vi "Execute.vi"(8 "Error In":errorcluster, 9 "Workspace":T1, 10 "Control In":T2, 11 "Dispense in":refnum<class "Dispense.lvclass">) -> (0 "Error Out":errorcluster, 2 "Control Out":T2, 3 "Dispense in 2":refnum<class "Dispense.lvclass">)   [LabVIEW 2020, in "Dispense.lvclass"]
uses:
  Dispense.lvclass
  Controller/Controllers.ctl
  Controller/I-O/I-O.lvclass
  Controller/Dispenser/Dispenser.lvclass
  C:/Program Files (x86)/Aerotech/A3200/LabVIEW/2010/Bin/Aerotech.A3200.dll
  Program Files (x86)/Aerotech/A3200/LabVIEW/2010/Bin/Aerotech.A3200.dll
  Workspace/Workspace.ctl
  Dispense.lvclass/Dispense.ctl
  Controller/Motion/Motion.lvclass
  Controller/Motion/A3200/A3200.lvclass
  Controller/Controller.lvclass
  Workspace/Fixture.lvclass
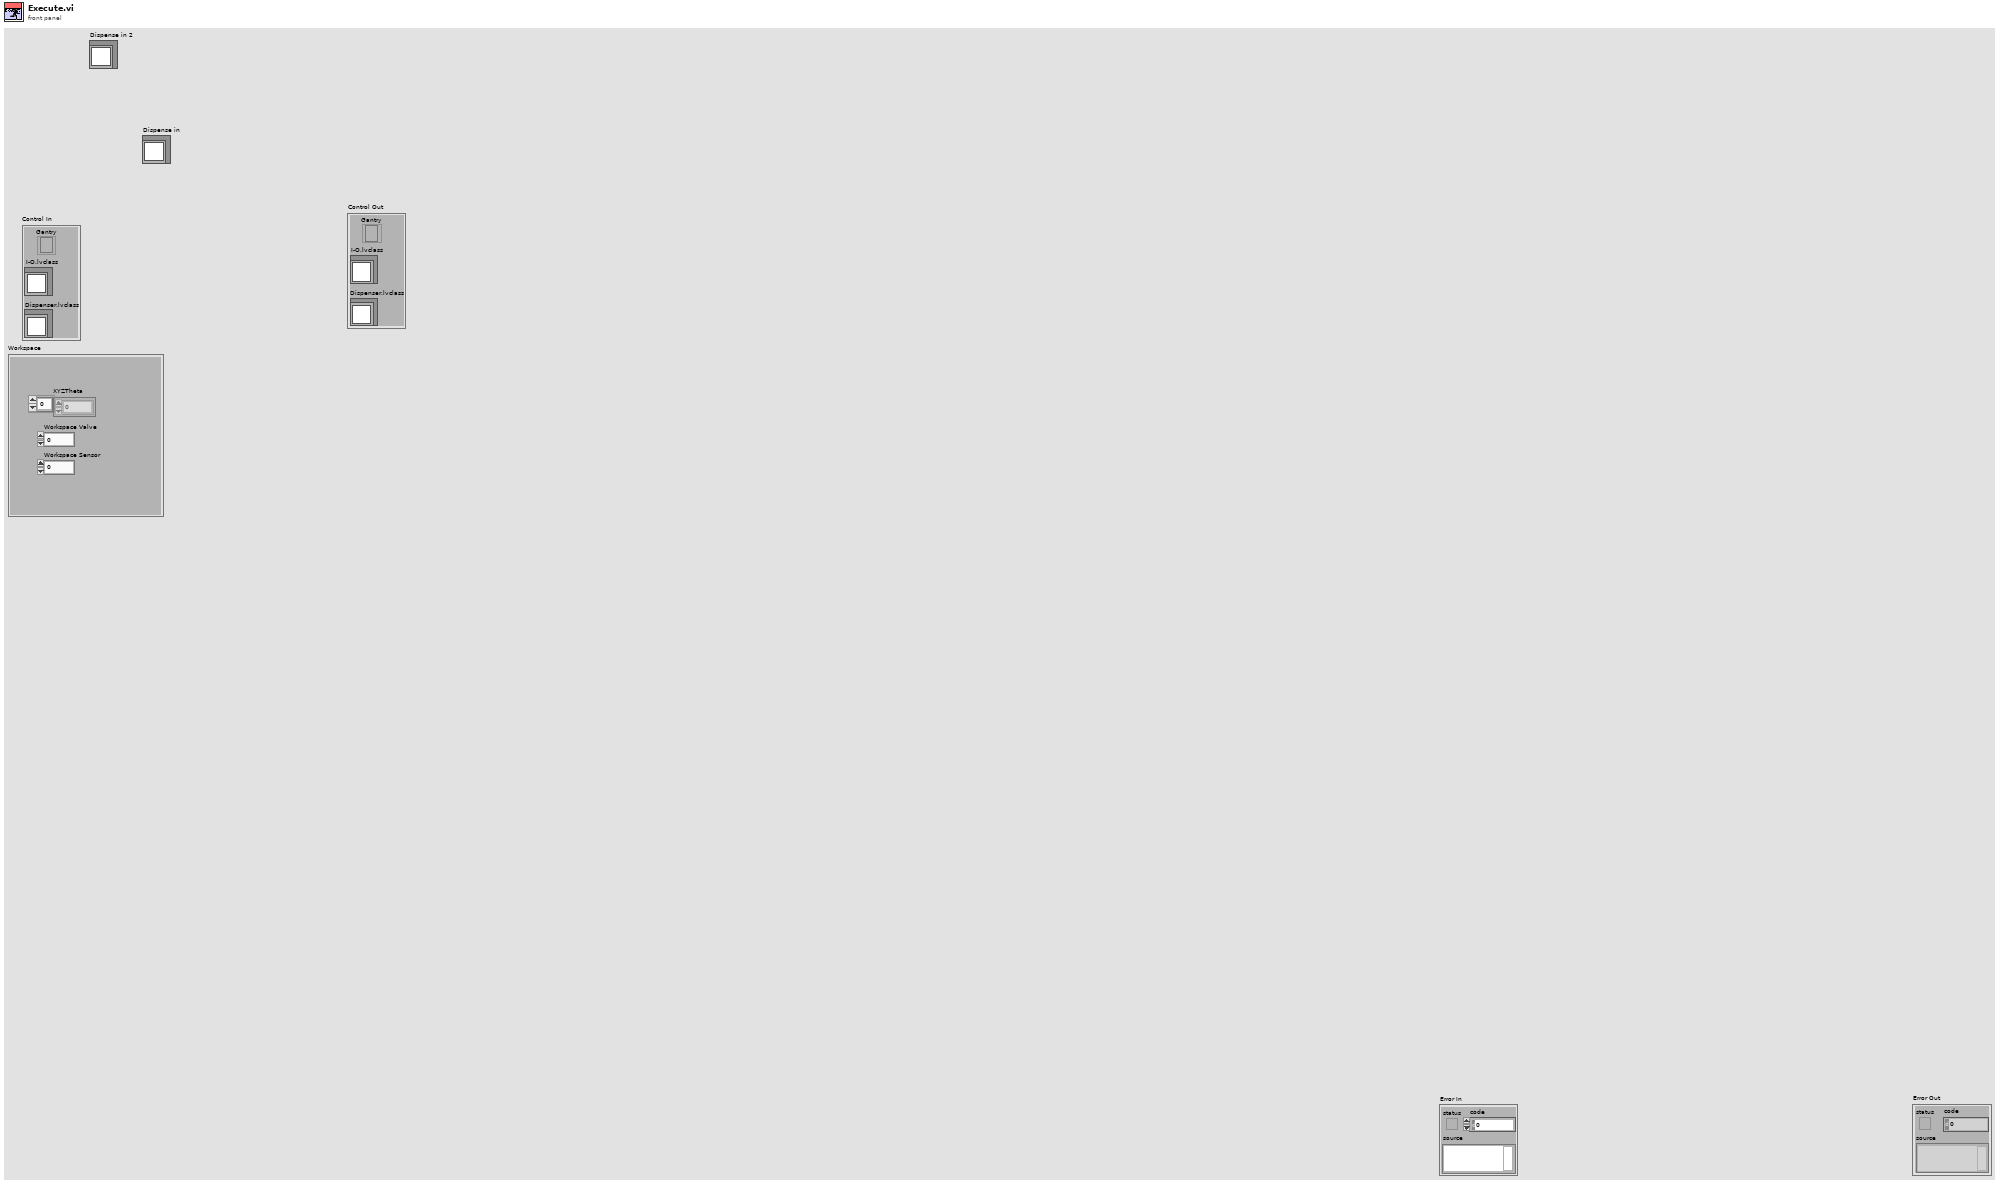
[diagram p1: front panel]
types:
  T1 = typedef "Fixture.lvclass/Workspace.ctl" = cluster{"XYZTheta":dbl[], "Workspace Valve":i32, "Workspace Sensor":i32}
  T2 = typedef "Controller.lvclass/Controllers.ctl" = cluster{"I-O.lvclass":refnum<class "I-O.lvclass">, "Dispenser.lvclass":refnum<class "Dispenser.lvclass">, "Gantry":refnum<k24>}
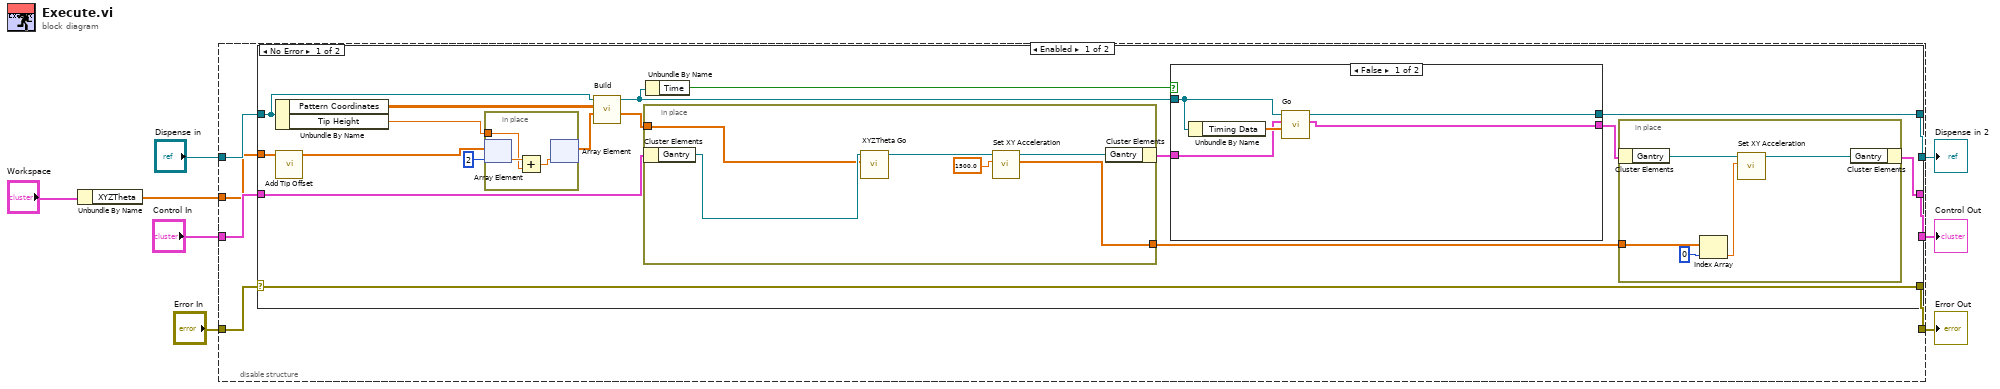
[diagram p0: block diagram]
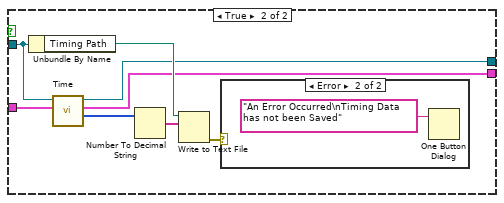
[diagram p2: hidden frame]
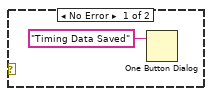
[diagram p3: hidden frame]
diagram:
  n1 = Unbundle By Name("Workspace") -> ("XYZTheta"=w2:dbl[])
  n2 = disable-structure shown="Enabled" {
    disable-tunnel: "Control In" -> [w15 w65]
    disable-tunnel: [w14 w65] -> w7
    disable-tunnel: "Dispense in" -> [w13 w67]
    disable-tunnel: "Error In" -> [w12 w66]
    disable-tunnel: [w11 w66] -> w4
    disable-tunnel: w2 -> [w10 _]
    disable-tunnel: [w9 w67] -> w1
    frame Enabled {
      n3 = case shown="No Error" w12 {
        selector: w12 -> [w32 w63]
        tunnel: w15 -> [w24 w64]
        tunnel: [w19 w64] -> w14
        tunnel: w13 -> [w23 w62]
        tunnel: [w32 w63] -> w11
        tunnel: w10 -> [w22 _]
        tunnel: [w30 w62] -> w9
        frame No Error {
          n4 = Unbundle By Name(w23) -> ("Pattern Coordinates"=w28:dbl[][], "Tip Height"=w25:dbl)
          n5 = call "Add Tip Offset.vi"("XYZTheta"=w22) -> ("XYZTheta"=w21:dbl[])  [unwired: 10 in]
          n6 = in-place {
            in-place-border: w25 -> [w53]
            n7 = in-place-array #1(w21, 2) -> (w55:dbl)
            n8 = Add(x=w55, y=w53) -> (x+y=w54:dbl)
            n9 = in-place-array #1(w54) -> (w26:dbl[])  [unwired: 1 out]
          }
          n10 = call-dynamic "Build.vi"("XYZTheta"=w26, "Pattern Coordinates"=w28, "Dispense in"=w23) -> ("Starting Coordinates"=w29:dbl[], "Dispense out"=w31:refnum<class "Dispense.lvclass">)  [unwired: 7 in]
          n11 = in-place {
            in-place-border: w29 -> [w56]
            in-place-border: [w58] -> w17
            n12 = in-place-cluster #2(w24) -> ("Gantry"=w61:refnum<k24>)
            n13 = call "XYZTheta Go.vi"("XYZTheta In"=w56, "Gantry 2"=w61) -> ("Gantry 3"=w60:refnum<k24>)  [unwired: 7 in, 2 out]
            n14 = call "Set XY Acceleration.vi"("mm/s"=1500.0, "Gantry 2"=w60) -> ("Array"=w58:dbl[], "Gantry 3"=w57:refnum<k24>)  [unwired: 7 in, 1 out]
            n15 = in-place-cluster #2("Gantry"=w57) -> (w20:T2)
          }
          n16 = Unbundle By Name(w31) -> ("Time"=w18:bool)
          n17 = case shown="False" w18 {
            tunnel: w31 -> [w39 w44]
            tunnel: w20 -> [w38 w46]
            tunnel: [w42 w45] -> w16
            tunnel: [w40 w43] -> w30
            frame False {
              n18 = Unbundle By Name(w39) -> ("Timing Data"=w41:dbl[])
              n19 = call-dynamic "Go.vi"("Timing Data"=w41, "Control In"=w38, "Dispense in"=w39) -> ("Control Out"=w42:T2, "Dispense Out"=w40:refnum<class "Dispense.lvclass">)  [unwired: 7 in]
            }
            frame True {
              n20 = Unbundle By Name(w44) -> ("Timing Path"=w48:path)
              n21 = call-dynamic "Time.vi"("Control In"=w46, "Dispense in"=w44) -> ("Timing Data"=w47:i32[], "Control Out"=w45:T2, "Dispense out"=w43:refnum<class "Dispense.lvclass">)  [unwired: 6 in, 1 out]
              n22 = Number To Decimal String(number=w47) -> (decimal integer string=w49:string[])  [unwired: 1 in]
              n23 = Write to Text File(file (use dialog)=w48, text=w49) -> (error out=w50:errorcluster)  [unwired: 2 in, 2 out]
              n24 = case shown="Error" w50 {
                frame No Error {
                  n25 = One Button Dialog(message="Timing Data Saved") -> ()  [unwired: 1 in, 1 out]
                }
                frame Error {
                  n26 = One Button Dialog(message="An Error Occurred\nTiming Data has not been Saved") -> ()  [unwired: 1 in, 1 out]
                }
              }
            }
          }
          n27 = in-place {
            in-place-border: w17 -> [w35]
            n28 = in-place-cluster #3(w16) -> ("Gantry"=w37:refnum<k24>)
            n29 = Index Array(array=w35, index=0) -> (element=w34:dbl)
            n30 = call "Set XY Acceleration.vi"("mm/s"=w34, "Gantry 2"=w37) -> ("Gantry 3"=w36:refnum<k24>)  [unwired: 7 in, 2 out]
            n31 = in-place-cluster #3("Gantry"=w36) -> (w19:T2)
          }
        }
        frame Error {
        }
      }
    }
    frame Disabled {
    }
  }
  "Control Out" <- w7
  "Error Out" <- w4
  "Dispense in 2" <- w1
